vi "解压缩.vi"(8 "error in (no error)":errorcluster caption="错误输入（无错误）", 11 "Zip file":path caption="Zip文件") -> (0 "error out":errorcluster, 2 "MD5":string, 3 "待校验的文件路径":path)   [LabVIEW 2016, in "数据传输系统-05.lvlib" / "update.lvlib"]
uses:
  update.lvlib
  <vilib>/zip/NI_Unzip.lvlib
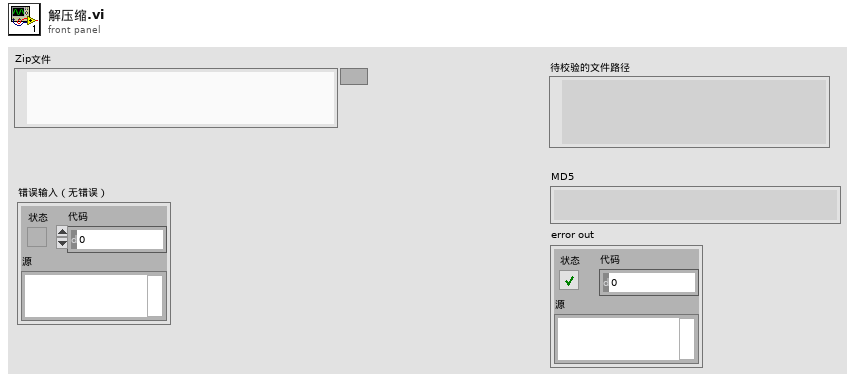
[diagram p1: front panel]
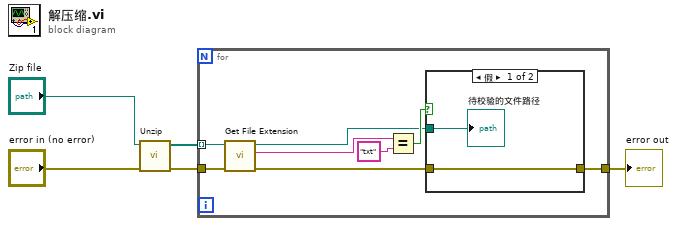
[diagram p0: block diagram]
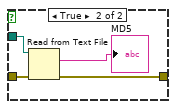
[diagram p2: hidden frame]
diagram:
  n1 = call <vilib>:"Unzip.vi"("error in (no error)"="error in (no error)", "Zip file"="Zip file") -> ("error out"=w3:errorcluster, "Unzipped files"=w4:path[])  [unwired: 7 in, 1 out]
  n2 = for {
    tunnel: w4 -> [w13] mode=indexing
    tunnel: w3 -> [w12]
    tunnel: [w6] -> w2
    n3 = call <vilib>:"Get File Extension.vi"("error in (no error)"=w12, "file"=w13) -> ("error out"=w7:errorcluster, "lowercase file extension"=w11:string, "dup file"=w8:path)  [unwired: 5 in, 2 out]
    n4 = Equal?(x=w11, y="txt") -> (x = y?=w9:bool)
    n5 = case shown="假" w9 {
      tunnel: w8 -> [w15 w19]
      tunnel: w7 -> [w14 w18]
      tunnel: [w14 w16] -> w6
      frame False {
        "待校验的文件路径" <- w15
      }
      frame True {
        n6 = Read from Text File(file (use dialog)=w19, error in=w18) -> (text=→"MD5":string, error out=w16:errorcluster)  [unwired: 2 in, 2 out]
      }
    }
  }
  "error out" <- w2
